vi "AdaptActivePowerToBMS.vi"(1 "p_sp":dbl, 2 "MaxChargePower":dbl, 3 "MaxDischargePower":dbl, 4 "Pdc Battery":dbl) -> (0 "p_sp Ok":dbl)   [LabVIEW 2017]
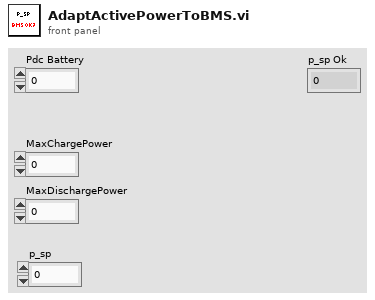
[diagram p1: front panel]
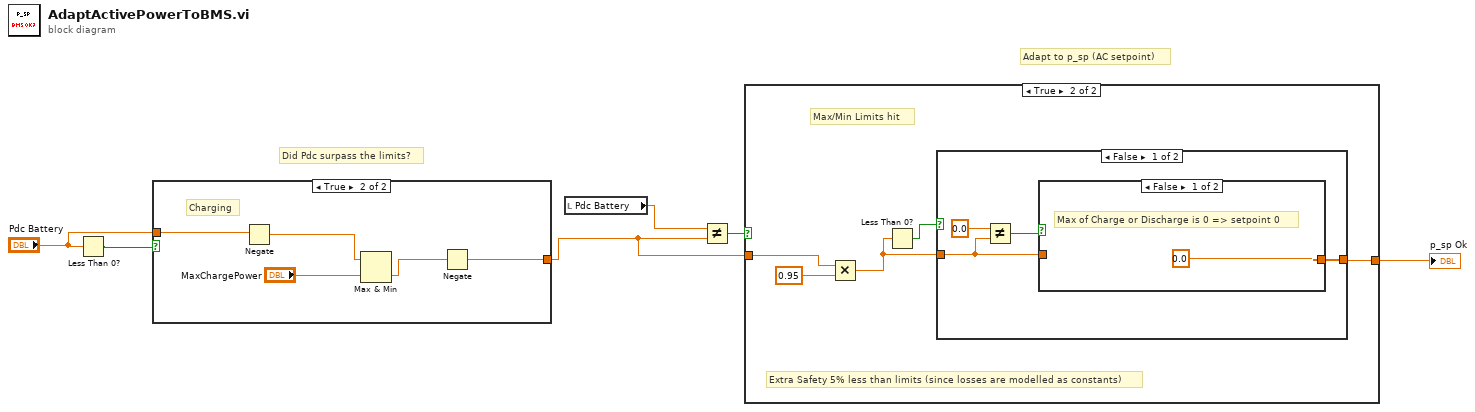
[diagram p0: block diagram]
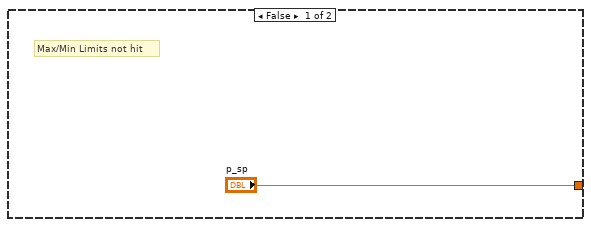
[diagram p2: hidden frame]
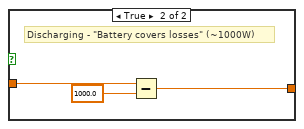
[diagram p3: hidden frame]
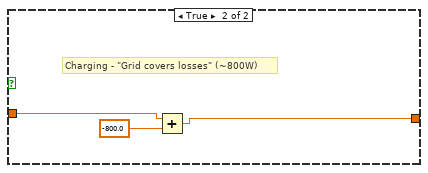
[diagram p4: hidden frame]
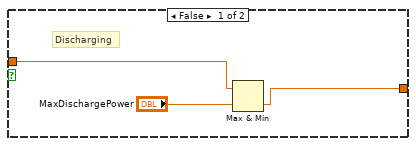
[diagram p5: hidden frame]
diagram:
  # "Did Pdc surpass the limits?"
  # "Adapt to p_sp (AC setpoint)"
  n1 = Less Than 0?(x="Pdc Battery") -> (x < 0?=w6:bool)
  n2 = case shown="True" w6 {
    tunnel: "Pdc Battery" -> [w8 w14]
    tunnel: [w7 w11] -> w1
    frame False {
      # "Discharging"
      n3 = Max & Min(x=w8, y="MaxDischargePower") -> (min(x,y)=w7:dbl)  [unwired: 1 out]
    }
    frame True {
      # "Charging"
      n4 = Negate(x=w14) -> (-x=w13:dbl)
      n5 = Max & Min(x=w13, y="MaxChargePower") -> (min(x,y)=w12:dbl)  [unwired: 1 out]
      n6 = Negate(x=w12) -> (-x=w11:dbl)
    }
  }
  n7 = local read "Pdc Battery"() -> (w3:dbl)
  n8 = Not Equal?(x=w3, y=w1) -> (x != y?=w2:bool)
  n9 = case shown="True" w2 {
    tunnel: ["p_sp" w19] -> w5
    tunnel: w1 -> [_ w18]
    frame False {
      # "Max/Min Limits not hit"
    }
    frame True {
      # "Extra Safety 5% less than limits (since losses are modelled as constants)"
      # "Max/Min Limits hit"
      n10 = Multiply(x=w18, y=0.95) -> (x*y=w16:dbl)
      n11 = Less Than 0?(x=w16) -> (x < 0?=w20:bool)
      n12 = case shown="False" w20 {
        tunnel: w16 -> [w22 w31]
        tunnel: [w24 w29] -> w19
        frame False {
          n13 = Not Equal?(x=0.0, y=w22) -> (x != y?=w23:bool)
          n14 = case shown="False" w23 {
            tunnel: w22 -> [_ w28]
            tunnel: [0.0 ("x") w26] -> w24
            frame False {
              # "Max of Charge or Discharge is 0 => setpoint 0"
            }
            frame True {
              # "Discharging - \"Battery covers losses\" (~1000W)"
              n15 = Subtract(x=w28, y=1000.0) -> (x-y=w26:dbl)
            }
          }
        }
        frame True {
          # "Charging - \"Grid covers losses\" (~800W)"
          n16 = Add(x=w31, y=-800.0) -> (x+y=w29:dbl)
        }
      }
    }
  }
  "p_sp Ok" <- w5
